vi "Filter2012Target.vi"(0 "Image In":T2, 1 "Red or Hue Range":cluster{"Lower value":i32, "Upper value":i32}={"Lower value"=80, "Upper value"=100}, 2 "Green or Sat Range":cluster{"Lower value":i32, "Upper value":i32}={"Lower value"=0, "Upper value"=255}, 3 "Blue or Luma or Val or Inten Range":cluster{"Lower value":i32, "Upper value":i32}={"Lower value"=20, "Upper value"=120}, 4 "Image Dst":T2) -> (5 "Image Out":T2, 6 "Blob Array":T1(array[cluster]), 7 "Lines Calibrated":T3(array[cluster]))   [LabVIEW 2011]
uses:
  <vilib>/vision/Image Controls.llb/IMAQ Image.ctl
  <vilib>/vision/NI_Vision_Development_Module.lvlib
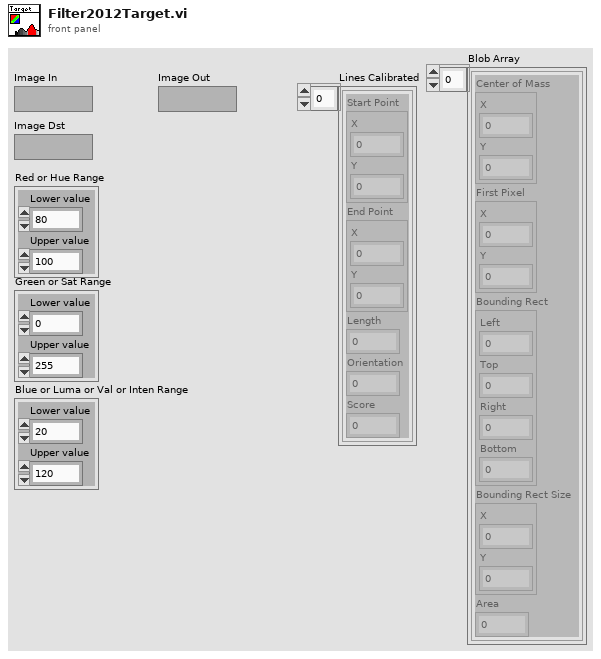
[diagram p1: front panel]
types:
  T1 = cluster{"Center of Mass":cluster{"X":dbl, "Y":dbl}, "First Pixel":cluster{"X":dbl, "Y":dbl}, "Bounding Rect":cluster{"Left":dbl, "Top":dbl, "Right":dbl, "Bottom":dbl}, "Bounding Rect Size":cluster{"X":dbl, "Y":dbl}, "Area":dbl}[]
  T2 = typedef "IMAQ Image.ctl" = refnum<image>
  T3 = cluster{"Start Point":cluster{"X":sgl, "Y":sgl}, "End Point":cluster{"X":sgl, "Y":sgl}, "Length":dbl, "Orientation":dbl, "Score":dbl}[]
  T4 = cluster{"Extraction Mode":u32, "Edge Threshold":i32, "Edge Filter Size":u32, "Min Length":i32, "Row Search Step Size":i32, "Col Search Step Size":i32, "Max Endpoint Gap":i32, "Closed":bool, "Subpixel":bool}
  T5 = cluster{"Rotation":bool, "Scale":bool, "Occlusion":bool, "Range Settings":cluster{"Match Constraints":u32, "Min":dbl, "Max":dbl}[]}
  T6 = cluster{"ID":enum32{"External", "Internal"}, "Type":u32, i32[]}
  T7 = cluster{"ID":enum32{"External", "Internal"}, "Type":u32, i32[]}[]
  T8 = cluster{i32[], cluster{"ID":enum32{"External", "Internal"}, "Type":u32, i32[]}[]}
  T9 = cluster{"Center of Mass":cluster{"X":dbl, "Y":dbl}, "First Pixel":cluster{"X":dbl, "Y":dbl}, "Bounding Rect":cluster{"Left":dbl, "Top":dbl, "Right":dbl, "Bottom":dbl}, "Bounding Rect Size":cluster{"X":dbl, "Y":dbl}, "Area":dbl}
  T10 = typedef "Particle Parameters" = i32
  T11 = cluster{"Start Point":cluster{"X":sgl, "Y":sgl}, "End Point":cluster{"X":sgl, "Y":sgl}, "Length":dbl, "Angle":dbl, "Score":dbl}[]
  T12 = cluster{"Particle Measurements (Pixels)[0]":dbl, "Particle Measurements (Pixels)[1]":dbl, "Particle Measurements (Pixels)[2]":dbl, "Particle Measurements (Pixels)[3]":dbl, "Particle Measurements (Pixels)[4]":dbl, "Particle Measurements (Pixels)[5]":dbl, "Particle Measurements (Pixels)[6]":dbl, "Particle Measurements (Pixels)[7]":dbl, "Particle Measurements (Pixels)[8]":dbl, "Particle Measurements (Pixels)[9]":dbl, "Particle Measurements (Pixels)[10]":dbl}
  T13 = cluster{"Particle Measurements (Pixels)[0]":dbl, "Particle Measurements (Pixels)[1]":dbl}
  T14 = cluster{"Particle Measurements (Pixels)[2]":dbl, "Particle Measurements (Pixels)[3]":dbl}
  T15 = cluster{"Particle Measurements (Pixels)[4]":dbl, "Particle Measurements (Pixels)[5]":dbl, "Particle Measurements (Pixels)[6]":dbl, "Particle Measurements (Pixels)[7]":dbl}
  T16 = cluster{"Particle Measurements (Pixels)[8]":dbl, "Particle Measurements (Pixels)[9]":dbl}
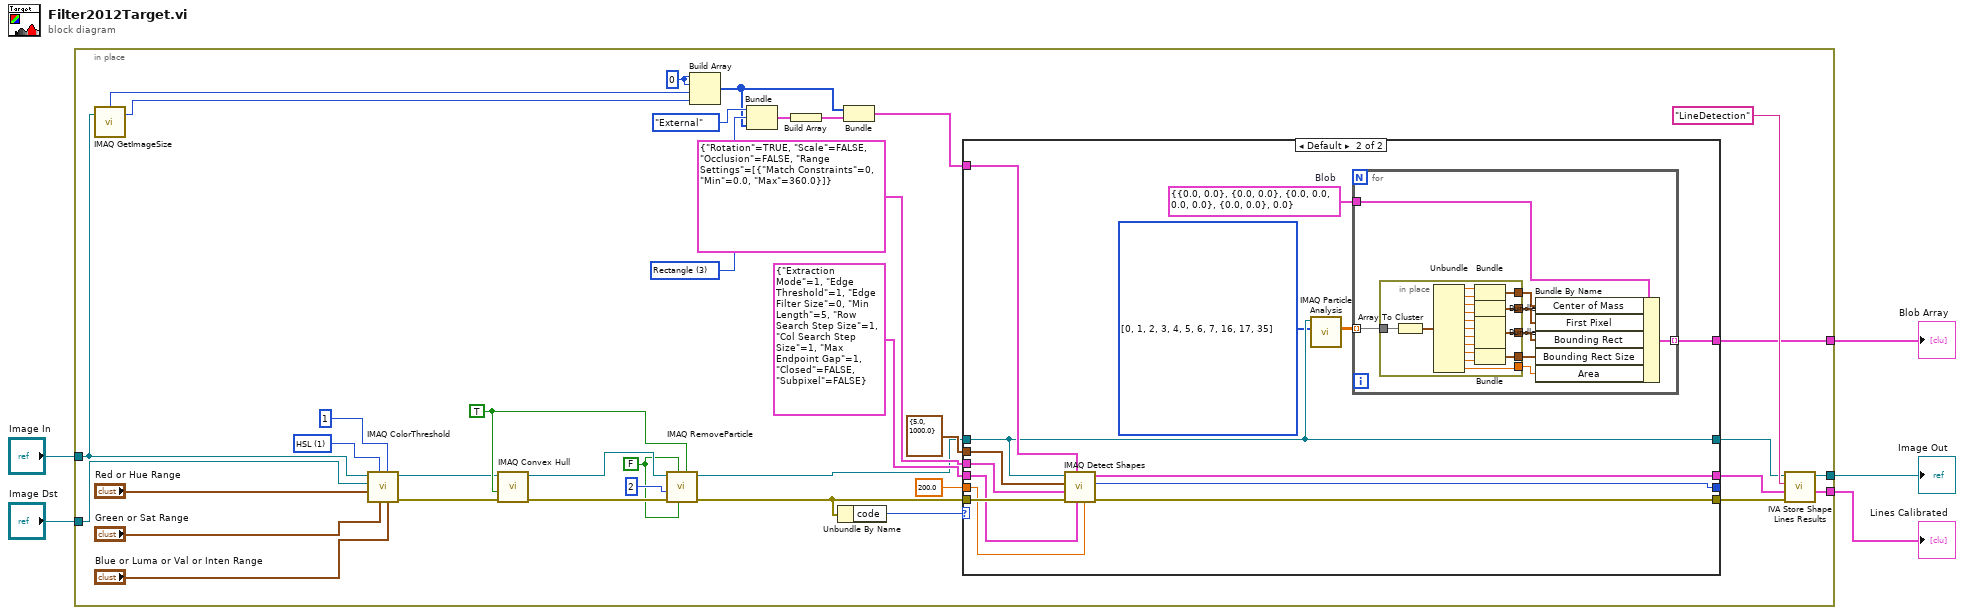
[diagram p0: block diagram]
diagram:
  n1 = in-place {
    in-place-border: "Image In" -> [w16]
    in-place-border: "Image Dst" -> [w27]
    in-place-border: [w26] -> w3
    in-place-border: [w10] -> w2
    in-place-border: [w9] -> w1
    w14 = 0 ("element")
    w15 = u32 3 items=["No Selection", "Point", "Line", "Rectangle", "Oval", "Polygon", "Freehand Region", "Annulus", "Unused2", "Unused3", "Broken Line", "Freehand Line", "Rotated Rectangle"] ("Type")
    w21 = TRUE ("Connectivity 4/8 (8)")
    w20 = FALSE ("Low Pass/High Pass (Low)")
    w41 = u16 1 items=["RGB", "HSL", "HSV", "HSI"] ("Color Mode")
    n2 = call "IMAQ GetImageSize"("Image"=w16) -> ("Y Resolution"=w12:i32, "X Resolution"=w13:i32)  [unwired: 3 in, 1 out]
    n3 = call "IMAQ ColorThreshold"("Blue or Luma or Val or Inten Range"="Blue or Luma or Val or Inten Range", "Replace Value"=1, "Green or Sat Range"="Green or Sat Range", "Color Mode"=w41, "Red or Hue Range"="Red or Hue Range", "Image Dst"=w27, "Image Src"=w16) -> ("error out"=w7:errorcluster, "Image Dst Out"=w8:T2)  [unwired: 1 in, 2 out]
    n4 = call "IMAQ Convex Hull"("error in (no error)"=w7, "Connectivity 4/8 (8)"=w21, "Image Src"=w8) -> ("error out"=w24:errorcluster, "Image Dst Out"=w25:T2)  [unwired: 1 in, 6 out]
    n5 = call "IMAQ RemoveParticle"("Connectivity 4/8 (8)"=w21, "Low Pass/High Pass (Low)"=w20, "Square/Hexa (Square)"=w20, "error in (no error)"=w24, "Number of Erosion"=2, "Image Src"=w25) -> ("error out"=w22:errorcluster, "Image Dst Out"=w23:T2)  [unwired: 1 in, 3 out]
    n6 = Build Array(w14, w14, w13, w12) -> (w6:i32[])
    n7 = Bundle("ID"=enum32{"External", "Internal"}."External", "Type"=w15, w6) -> (w11:T6)  [unwired: 1 in]
    n8 = Build Array(w11) -> (w18:T7)
    n9 = Unbundle By Name(w22) -> ("code"=w29:i32)
    n10 = Bundle(w6, w18) -> (w19:T8)  [unwired: 1 in]
    n11 = case shown="Default" w29 {
      tunnel: w22 -> [_ w57]
      tunnel: [_ w56] -> _
      tunnel: T5 {"Rotation"=TRUE, "Scale"=FALSE, "Occlusion"=FALSE, "Range Settings"=[{"Match Constraints"=0, "Min"=0.0, "Max"=360.0}]} ("Match Options") -> [_ w55]
      tunnel: T4 {"Extraction Mode"=1, "Edge Threshold"=1, "Edge Filter Size"=0, "Min Length"=5, "Row Search Step Size"=1, "Col Search Step Size"=1, "Max Endpoint Gap"=1, "Closed"=FALSE, "Subpixel"=FALSE} ("Curve Parameters") -> [_ w54]
      tunnel: 200.0 ("Minimum match score") -> [_ w53]
      tunnel: cluster{"Min Radius":dbl, "Max Radius":dbl} {"Min Radius"=5.0, "Max Radius"=1000.0} ("Line Descriptor") -> [_ w52]
      tunnel: w19 -> [_ w51]
      tunnel: w23 -> [w43 w48]
      tunnel: [_ w50] -> w31
      tunnel: [_ w49] -> w30
      tunnel: [w43 w48] -> w28
      tunnel: [_ w44] -> w9
      frame -1074396199, -1074396198 {
        # "Discard Coordinate\nSystem Error"
      }
      frame Default {
        w45 = T9 {"Center of Mass"={"X"=0.0, "Y"=0.0}, "First Pixel"={"X"=0.0, "Y"=0.0}, "Bounding Rect"={"Left"=0.0, "Top"=0.0, "Right"=0.0, "Bottom"=0.0}, "Bounding Rect Size"={"X"=0.0, "Y"=0.0}, "Area"=0.0}  # Blob
        w47 = T10[] [0, 1, 2, 3, 4, 5, 6, 7, 16, 17, 35] items=["Center of Mass X", "Center of Mass Y", "First Pixel X", "First Pixel Y", "Bounding Rect Left", "Bounding Rect Top", "Bounding Rect Right", "Bounding Rect Bottom", "Max Feret Diameter Start X", "Max Feret Diameter Start Y", "Max Feret Diameter End X", "Max Feret Diameter End Y", "Max Horiz. Segment Length Left", "Max Horiz. Segment Length Right", "Max Horiz. Segment Length Row", "-", "Bounding Rect Width", "Bounding Rect Height", "Bounding Rect Diagonal", "Perimeter", "Convex Hull Perimeter", "Holes' Perimeter", "Max Feret Diameter", "Equivalent Ellipse Major Axis", "Equivalent Ellipse Minor Axis", "Equivalent Ellipse Minor Axis (Feret)", "Equivalent Rect Long Side", "Equivalent Rect Short Side", "Equivalent Rect Diagonal", "Equivalent Rect Short Side (Feret)", "Average Horiz. Segment Length", "Average Vert. Segment Length", "Hydraulic Radius", "Waddel Disk Diameter", "-", "Area", "Holes' Area", "Particle & Holes' Area", "Convex Hull Area", "Image Area", "-", "Number of Holes", "Number of Horiz. Segments", "Number of Vert. Segments", "-", "Orientation", "Max Feret Diameter Orientation", "-", "% Area/Image Area", "% Area/(Particle & Holes' Area)", "Ratio of Equivalent Ellipse Axes", "Ratio of Equivalent Rect Sides", "-", "Elongation Factor", "Compactness Factor", "Heywood Circularity Factor", "Type Factor", "-", "Sum X", "Sum Y", "Sum XX", "Sum XY", "Sum YY", "Sum XXX", "Sum XXY", "Sum XYY", "Sum YYY", "-", "Moment of Inertia XX", "Moment of Inertia XY", "Moment of Inertia YY", "Moment of Inertia XXX", "Moment of Inertia XXY", "Moment of Inertia XYY", "Moment of Inertia YYY", "Norm. Moment of Inertia XX", "Norm. Moment of Inertia XY", "Norm. Moment of Inertia YY", "Norm. Moment of Inertia XXX", "Norm. Moment of Inertia XXY", "Norm. Moment of Inertia XYY", "Norm. Moment of Inertia YYY", "Hu Moment 1", "Hu Moment 2", "Hu Moment 3", "Hu Moment 4", "Hu Moment 5", "Hu Moment 6", "Hu Moment 7"] ("Pixel Measurements")
        n12 = call-poly "IMAQ Detect Shapes"("Minimum match score"=w53, "Curve Parameters"=w54, "ROI Descriptor"=w51, "error in (no error)"=w57, "Match Options"=w55, "Line Descriptor"=w52, "Image"=w48) -> ("error out"=w49:errorcluster, "Number of Matches Returned"=w56:i32, "Lines"=w50:T11)  [unwired: 2 out]
        n13 = call "IMAQ Particle Analysis"("Pixel Measurements"=w47, "Image"=w48) -> ("Particle Measurements (Pixels)"=w46:dbl[][])  [unwired: 4 in, 5 out]
        n14 = for {
          tunnel: w46 -> [w65] mode=indexing
          tunnel: w45 -> [w64]
          tunnel: [w58] -> w44 mode=indexing
          n15 = in-place {
            in-place-border: w65 -> [w82]
            in-place-border: [w70] -> w63
            in-place-border: [w69] -> w62
            in-place-border: [w68] -> w61
            in-place-border: [w67] -> w60
            in-place-border: [w66] -> w59
            n16 = Array To Cluster(array=w82) -> (cluster=w81:T12)
            n17 = Unbundle(w81) -> ("Particle Measurements (Pixels)[0]"=w80:dbl, "Particle Measurements (Pixels)[1]"=w79:dbl, "Particle Measurements (Pixels)[2]"=w78:dbl, "Particle Measurements (Pixels)[3]"=w77:dbl, "Particle Measurements (Pixels)[4]"=w76:dbl, "Particle Measurements (Pixels)[5]"=w75:dbl, "Particle Measurements (Pixels)[6]"=w74:dbl, "Particle Measurements (Pixels)[7]"=w73:dbl, "Particle Measurements (Pixels)[8]"=w72:dbl, "Particle Measurements (Pixels)[9]"=w71:dbl, "Particle Measurements (Pixels)[10]"=w66:dbl)
            n18 = Bundle("Particle Measurements (Pixels)[0]"=w80, "Particle Measurements (Pixels)[1]"=w79) -> (w70:T13)  [unwired: 1 in]
            n19 = Bundle("Particle Measurements (Pixels)[2]"=w78, "Particle Measurements (Pixels)[3]"=w77) -> (w69:T14)  [unwired: 1 in]
            n20 = Bundle("Particle Measurements (Pixels)[4]"=w76, "Particle Measurements (Pixels)[5]"=w75, "Particle Measurements (Pixels)[6]"=w74, "Particle Measurements (Pixels)[7]"=w73) -> (w68:T15)  [unwired: 1 in]
            n21 = Bundle("Particle Measurements (Pixels)[8]"=w72, "Particle Measurements (Pixels)[9]"=w71) -> (w67:T16)  [unwired: 1 in]
          }
          n22 = Bundle By Name(cluster=w64, "Center of Mass"=w63, "First Pixel"=w62, "Bounding Rect"=w61, "Bounding Rect Size"=w60, "Area"=w59) -> (w58:T9)
        }
      }
    }
    n23 = call <vilib>:"IVA Store Shape Lines Results.vi"("error in (no error)"=w30, "Lines"=w31, "Step Name"="LineDetection", "Image in"=w28) -> ("Lines Calibrated"=w26:T3, "Image dup"=w10:T2)  [unwired: 6 out]
  }
  "Lines Calibrated" <- w3
  "Image Out" <- w2
  "Blob Array" <- w1
